vi "Test API Execution from Test Case.vi"(8 "error in (no error)":errorcluster, 11 "API Test in":refnum<class "API Test.lvclass">) -> (0 "error out":errorcluster, 3 "API Test out":refnum<class "API Test.lvclass">)   [LabVIEW 2020, in "LUnit Tests.lvlib" / "API Test.lvclass"]
uses:
  API Test.lvclass
  C:/Program Files (x86)/National Instruments/LabVIEW 2020/vi.lib/Asteme/LUnit/Test Case.lvclass
  source/Examples/Basic Example/Dummy/Dummy.lvclass
  C:/Users/anton/Documents/GitHub/LUnit/source/Framework/Test Case/LUnit Test Case.lvclass
  <vilib>/Asteme/LUnit/Test Case.lvclass/Test Case.ctl
  <vilib>/Asteme/LUnit/LUnit Assertion Result.lvclass/LUnit Assertion Result.ctl
  <vilib>/Asteme/LUnit/LUnit Test Case Result.lvclass/LUnit Test Case Result.ctl
  <vilib>/Asteme/LUnit/LUnit Method Result.lvclass/LUnit Method Result.ctl
  <vilib>/Asteme/LUnit/Palette/Fail.vi
  <vilib>/Asteme/LUnit/Palette/Pass.vi
  <vilib>/Asteme/LUnit/Set Assertion Type.vi
  <vilib>/Asteme/LUnit/Add test result.vi
  <vilib>/Asteme/LUnit/LUnit Write Passed.vi
  <vilib>/Asteme/LUnit/LUnit Write Message.vi
  <vilib>/Asteme/LUnit/LUnit Write Description.vi
  <vilib>/Asteme/LUnit/LUnit Write Assertion Type.vi
  <vilib>/Asteme/LUnit/LUnit Record Assertion Result.vi
  <vilib>/Asteme/LUnit/LUnit Aggregate Assertion Results.vi
  <vilib>/Asteme/LUnit/Assertion Result/LUnit Read Status.vi
  <vilib>/Asteme/LUnit/LUnit Read Message.vi
  <vilib>/Asteme/LUnit/LUnit Read Description.vi
  <vilib>/Asteme/LUnit/Method Result/LUnit Merge Status.vi
  <vilib>/Asteme/LUnit/LUnit Concatenate result strings.vi
  <vilib>/Asteme/LUnit/LUnit Assertion Result.lvclass
  source/Framework/Execution API/Execution API.lvclass
  <vilib>/Asteme/LUnit/Test Case.lvclass
  C:/Users/anton/Documents/GitHub/LUnit/tests/API Test/API Test.lvclass
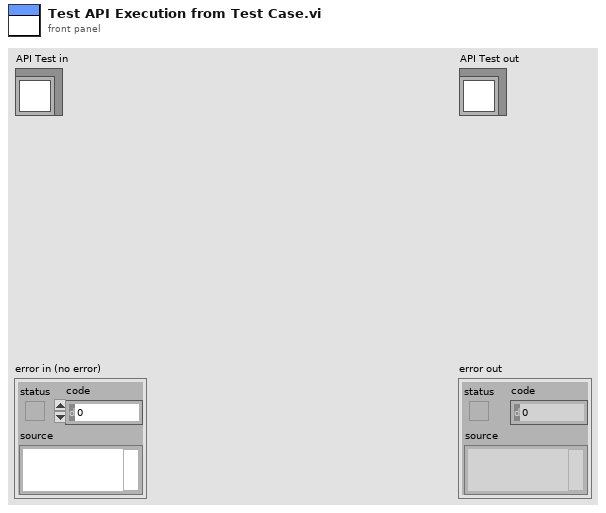
[diagram p1: front panel]
types:
  T1 = cluster{"Event Registration Refnum":refnum<event-registration>, "Event Registration Refnum":refnum<event-registration>}
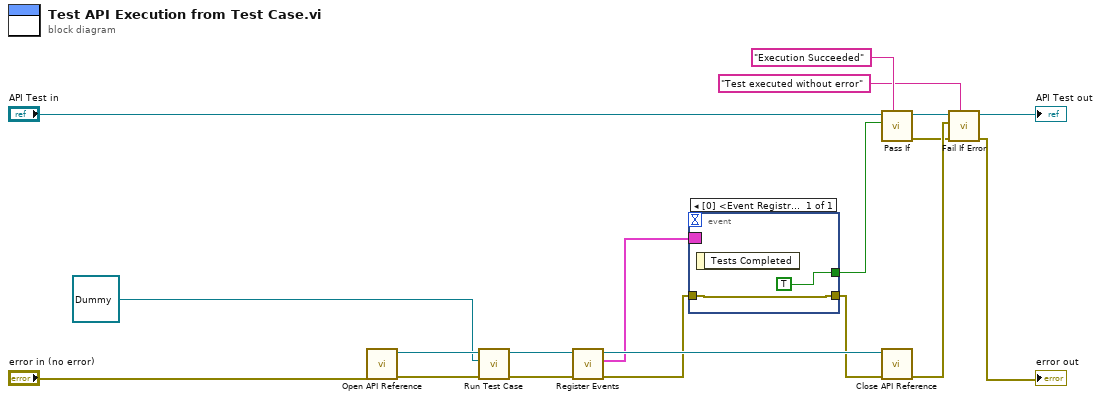
[diagram p0: block diagram]
diagram:
  n1 = call "Open API Reference.vi"("error in (no error)"="error in (no error)") -> ("error out"=w2:errorcluster, "Execution API out"=w5:refnum<class "Execution API.lvclass">)  [unwired: 9 in]
  n2 = call "Run Test Case.vi"("error in (no error)"=w2, "Test Case"=refnum<class "Dummy.lvclass"> refnum ("Dummy.lvclass"), "Execution API In"=w5) -> ("error out"=w3:errorcluster, "Execution API Out"=w4:refnum<class "Execution API.lvclass">)  [unwired: 7 in]
  n3 = call "Register Events.vi"("error in (no error)"=w3, "Execution API In"=w4) -> ("error out"=w7:errorcluster, "Result Events"=w14:T1, "Execution API Out"=w19:refnum<class "Execution API.lvclass">)  [unwired: 7 in]
  n4 = event shown="[0] <Event Registration Refnum.Test Completed>: User Event" {
    selector: w14 -> [_]
    dyn-events: _ -> [_]
    timeout: _ -> [_]
    tunnel: [TRUE] -> w11
    tunnel: [w20] -> w6
    tunnel: w7 -> [w20]
    event User Event {
      n5 = event-data() -> ()  [unwired: 1 in, 1 out]
    }
  }
  n6 = call <vilib>:"Pass If.vi"("Description"="Execution Succeeded", "Pass?"=w11, "LUnit Test Case In"="API Test in") -> ("error out"=w12:errorcluster, "LUnit Test Case Out"=w13:refnum<class "API Test.lvclass">)  [unwired: 7 in]
  n7 = call "Close API Reference.vi"("error in (no error)"=w6, "Execution API in"=w19) -> ("error out"=w16:errorcluster)  [unwired: 9 in]
  n8 = call <vilib>:"Fail If Error.vi"("Description"="Test executed without error", "error in (no error)"=w12, "Assert error"=w16, "LUnit Test Case In"=w13) -> ("error out"=→"error out":errorcluster, "LUnit Test Case Out"=→"API Test out":refnum<class "API Test.lvclass">)  [unwired: 6 in]
